vi "GetValue.vi"(0 "reference":refnum<vi>, 1 "Input":string, 3 "error in (no error)":errorcluster) -> (7 "Answer":string, 9 "Found?":bool, 10 "error out":errorcluster)   [LabVIEW 2019]
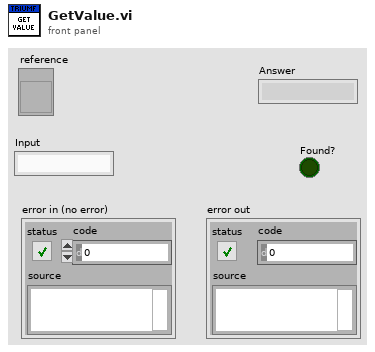
[diagram p1: front panel]
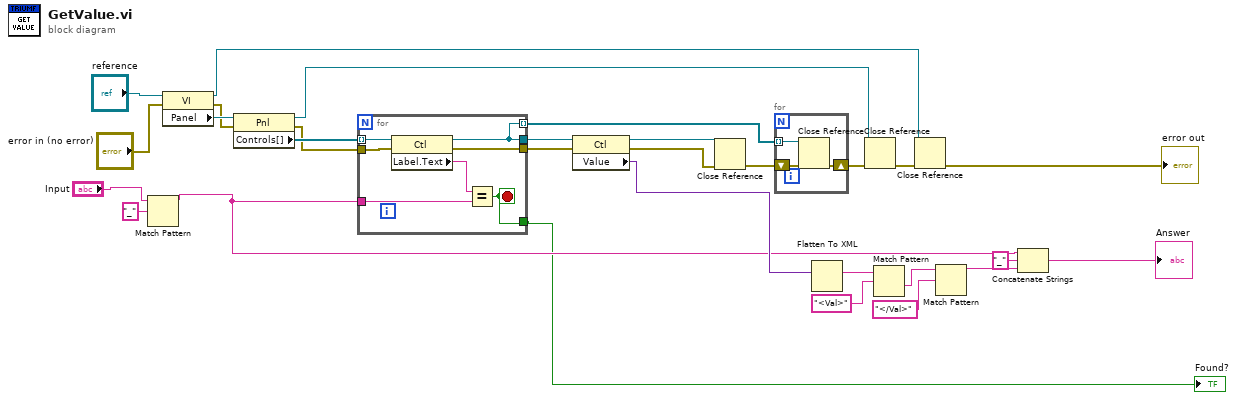
[diagram p0: block diagram]
diagram:
  n1 = Match Pattern(string="Input", regular expression="_") -> (before substring=w12:string)  [unwired: 1 in, 3 out]
  n2 = property class="VI"(reference="reference", error in="error in (no error)") -> (reference out=w29:refnum<vi>, error out=w25:errorcluster, "Panel"=w26:refnum<vi>)
  n3 = property class="Pnl"(reference=w26, error in=w25) -> (reference out=w28:refnum<vi>, error out=w3:errorcluster, "Controls[]"=w4:refnum<vi>[])
  n4 = for {
    tunnel: w4 -> [w36] mode=indexing
    tunnel: [w35] -> w7 mode=indexing
    tunnel: [w35] -> w8
    tunnel: [w34] -> w5
    tunnel: w12 -> [w33]
    tunnel: w3 -> [w31]
    tunnel: [w30] -> w11
    stop <- w30 stop-if-true
    n5 = property class="Ctl"(reference=w36, error in=w31) -> (reference out=w35:refnum<vi>, error out=w34:errorcluster, "Label.Text"=w32:string)
    n6 = Equal?(x=w32, y=w33) -> (x = y?=w30:bool)
  }
  "Found?" <- w11
  n7 = property class="Ctl"(reference=w8, error in=w5) -> (reference out=w10:refnum<vi>, error out=w9:errorcluster, "Value"=w18:variant)
  n8 = Close Reference(reference=w10, error in (no error)=w9) -> (error out=w6:errorcluster)
  n9 = for {
    tunnel: w7 -> [w39] mode=indexing
    shift-right: [w38] -> w2
    shift-left: w6 -> [w37]
    n10 = Close Reference(reference=w39, error in (no error)=w37) -> (error out=w38:errorcluster)
  }
  n11 = Flatten To XML(anything=w18) -> (xml string=w21:string)
  n12 = Close Reference(reference=w28, error in (no error)=w2) -> (error out=w27:errorcluster)
  n13 = Match Pattern(string=w21, regular expression="<Val>") -> (after substring=w22:string)  [unwired: 1 in, 3 out]
  n14 = Close Reference(reference=w29, error in (no error)=w27) -> (error out=→"error out":errorcluster)
  n15 = Match Pattern(string=w22, regular expression="</Val>") -> (before substring=w16:string)  [unwired: 1 in, 3 out]
  n16 = Concatenate Strings(w12, "_" ("string"), w16) -> (→"Answer":string)
